vi "禹山溶解氧校准.vi"() -> ()   [LabVIEW 2016, in "斯坦道多参数.lvlib"]
uses:
  <vilib>/Utility/miscctls.llb/LVPointTypeDef.ctl
  <vilib>/Analysis/NI_AALBase.lvlib
  <vilib>/Analysis/NI_AALPro.lvlib
  <vilib>/Utility/config.llb/NI_LVConfig.lvlib
panel:
  out "滤波设定":dbl
  out "第二点信号值":dbl
  out "第一点信号值":dbl
  out "通讯状态":string
  in  "盐度自动获取":bool
  in  "大气压补偿":dbl format="%#.2f"
  in  "盐度补偿":dbl format="%#.2f"
  out "DO %":dbl caption="饱和度值" format="%#.2f"
  out "第二点校准值":dbl
  out "第一点校准值":dbl
  out "最小值":sgl format="%.2g"
  out "最大值":sgl format="%.2g"
  in  "校准停止":bool
  in  "校准模式":u16(ring) items=["两点校准", "单点校准"]
  in  "标液2":dbl
  in  "标液1":dbl
  out "波形图表":dbl(graph) caption="历史曲线"
  out "温度测量值":dbl caption="温度" format="%#.2f"
  out "变异系数":dbl format="%.6g"
  out "standard deviation":dbl caption="标准差" format="%0.2f"
  out "mean":dbl caption="均值" format="%0.2f"
  out "提示":string
  in  "校准启动":bool
  out "DO mg/L":dbl caption="测试值" format="%#.2f"
  out "电极斜率":dbl format="%#.6f"
  out "电极零点":dbl format="%#.6f"
  # "溶解氧电极设定"
  # "℃"
  # "%"
  # "mg/L"
  # "kPa"
  # "请选择校准模式:"
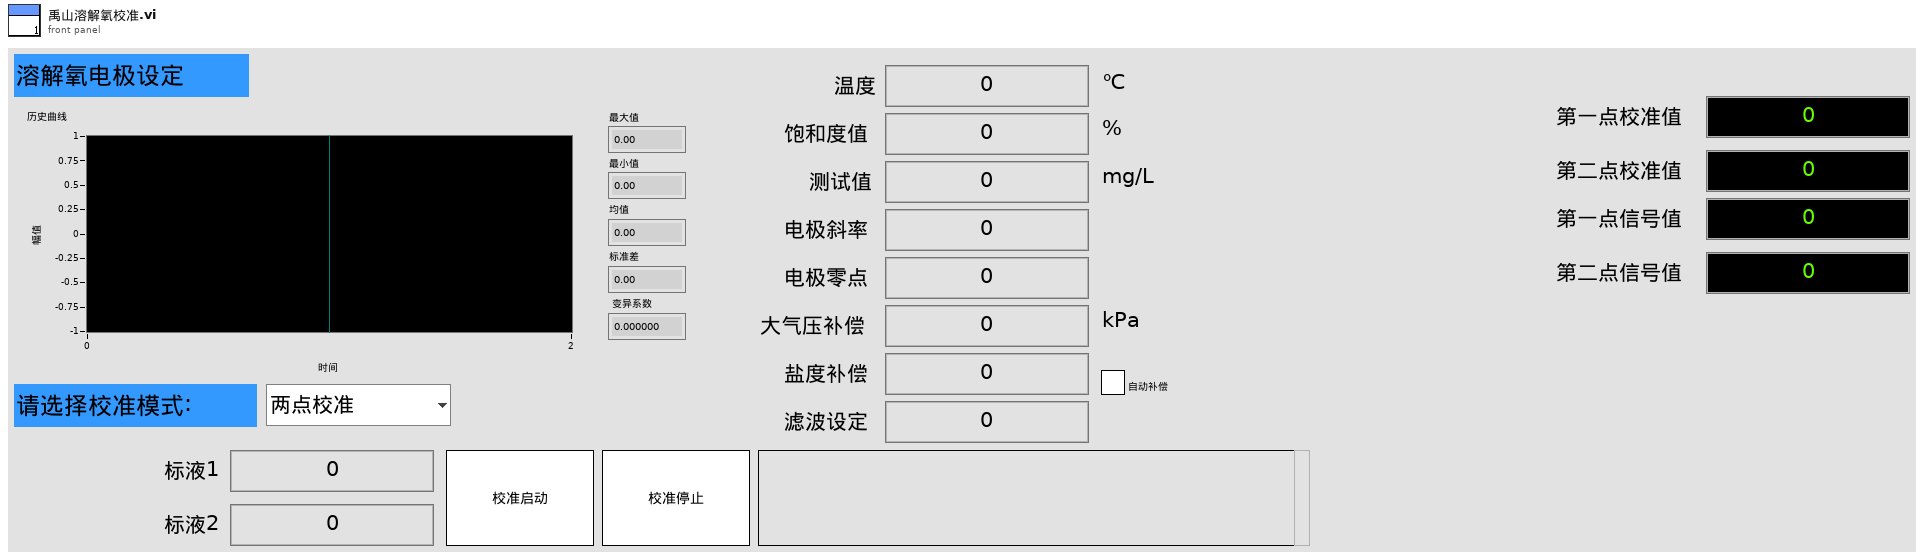
[diagram p1: front panel]
types:
  T1 = enum16{"pH", "DO", "Cond", "Turb", "ORP", "叶绿素a", "藻密度"}
  T2 = typedef "LVPointTypeDef.ctl" = cluster{"Horizontal":i16, "Vertical":i16}
  T3 = cluster{"pH":u32, "DO":u32, "Cond":u32, "Turb":u32, "叶绿素a":u32, "藻密度":u32, "ORP":u32}
  T4 = typedef "NI_LVConfig.lvlib/Config Data RefNum.ctl" = refnum<k1>
  T5 = enum8{"Enabled", "Disabled", "Disabled and Grayed Out"}
  T6 = cluster{"ph":bool, "DO":bool, "Cond":bool, "Turb":bool, "叶绿素a":bool, "藻密度":bool, "ORP":bool}
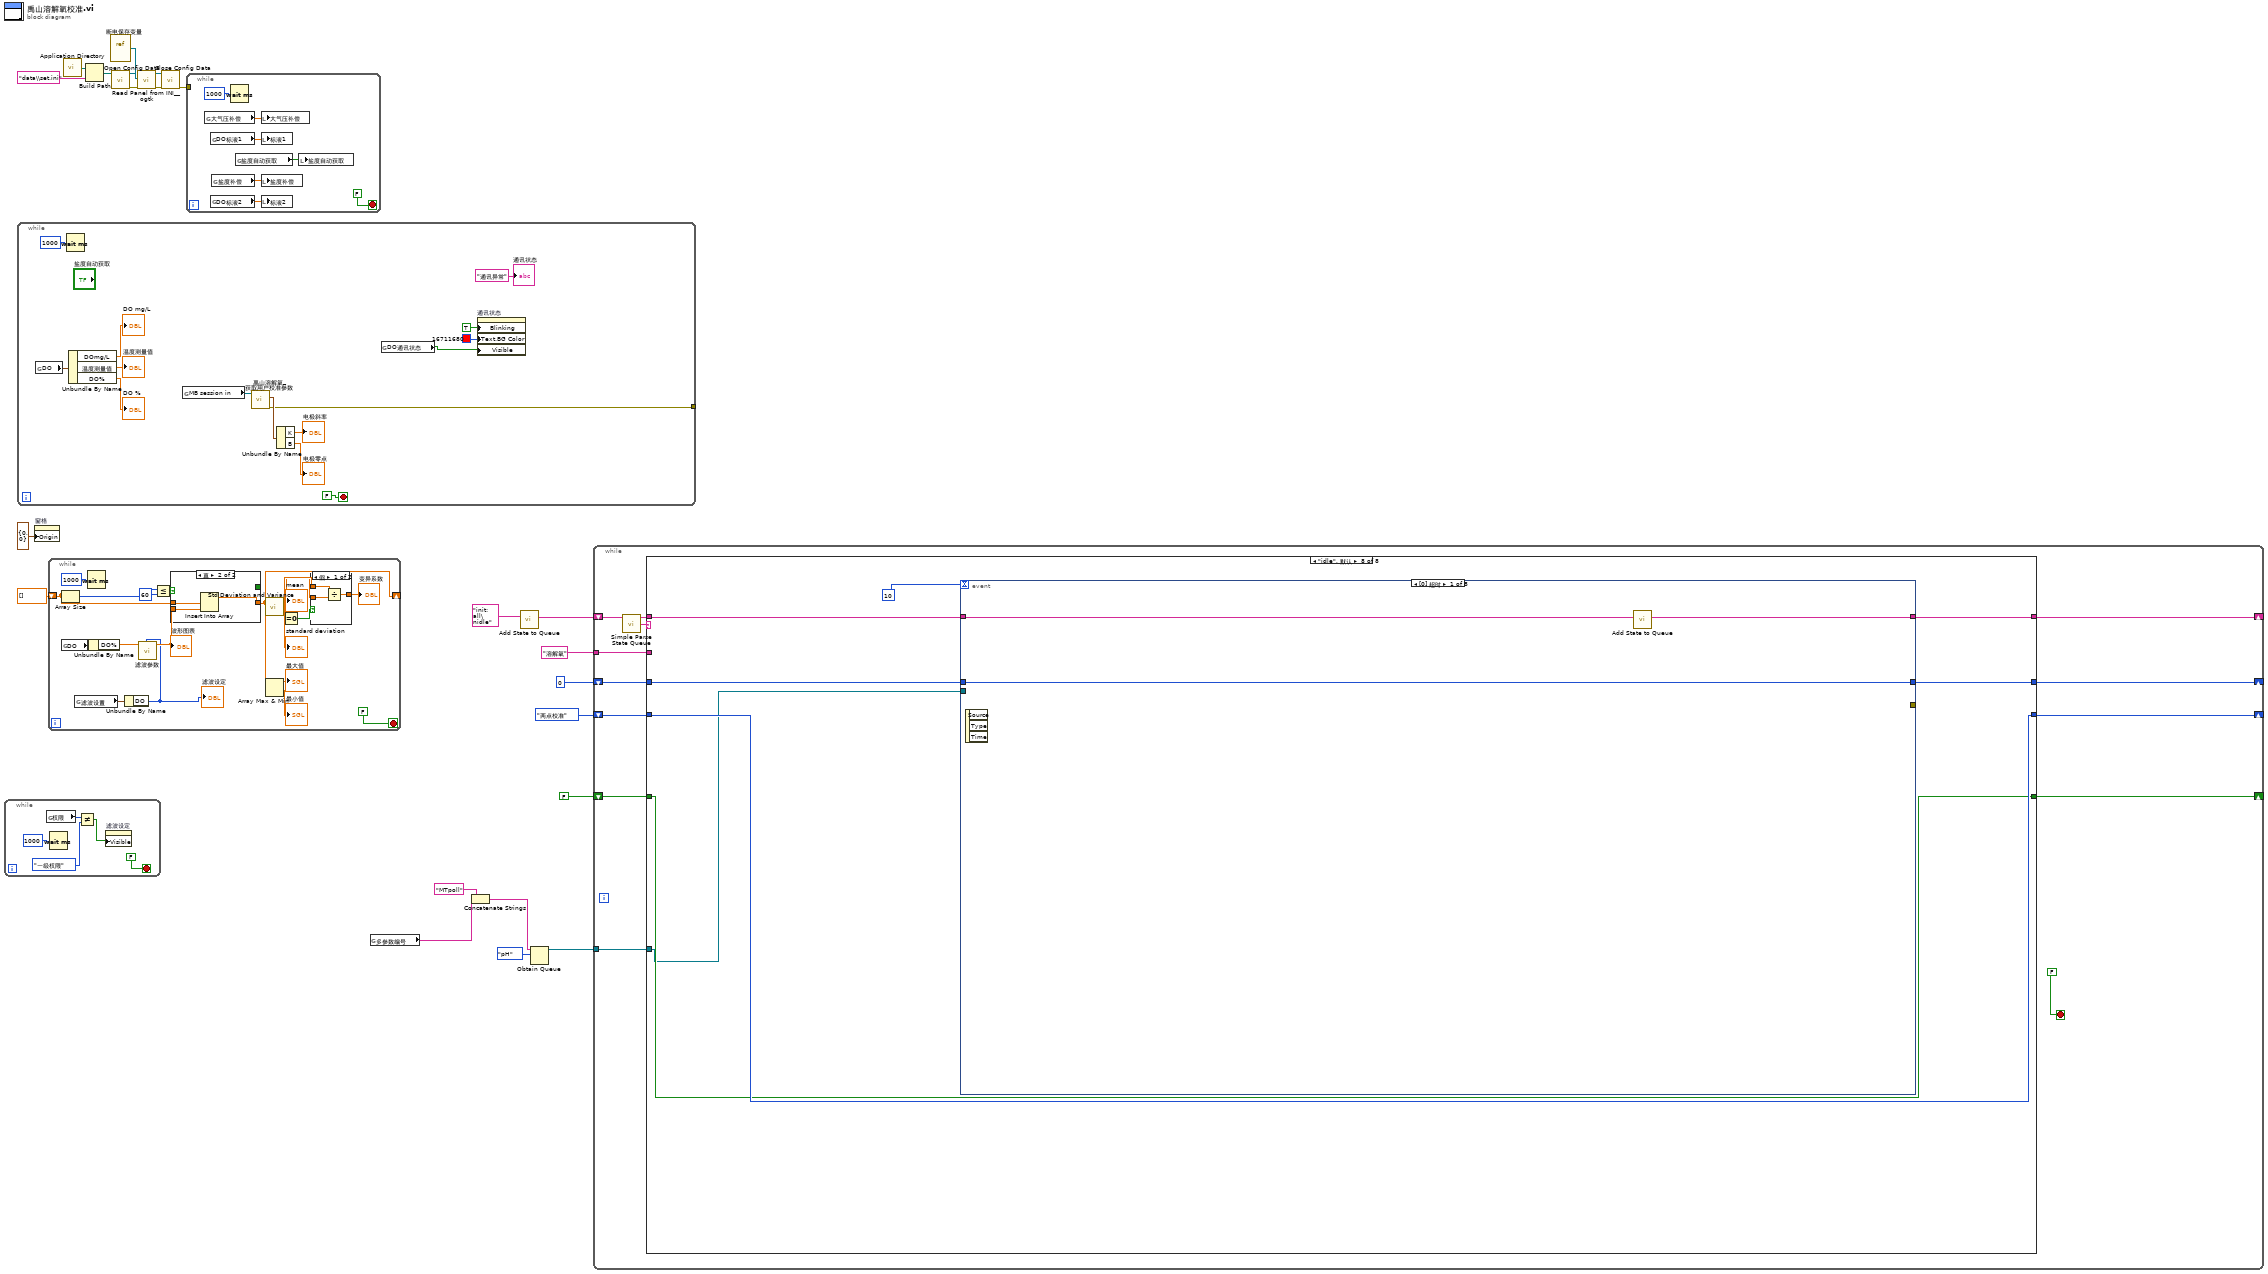
[diagram p0: block diagram]
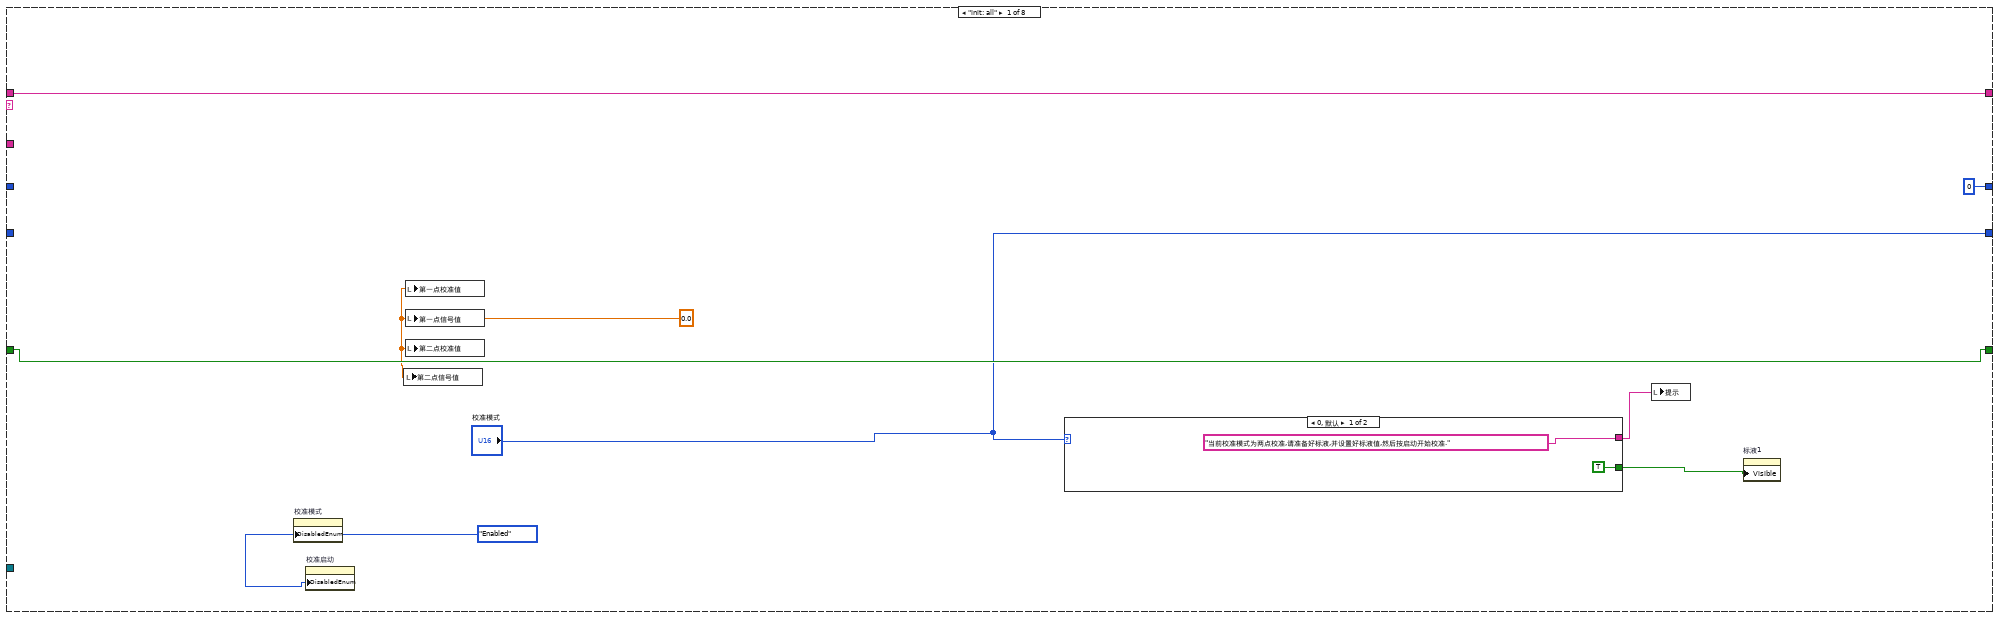
[diagram p2: hidden frame]
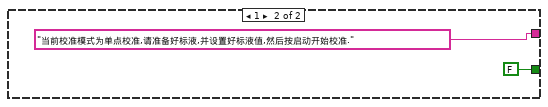
[diagram p3: hidden frame]
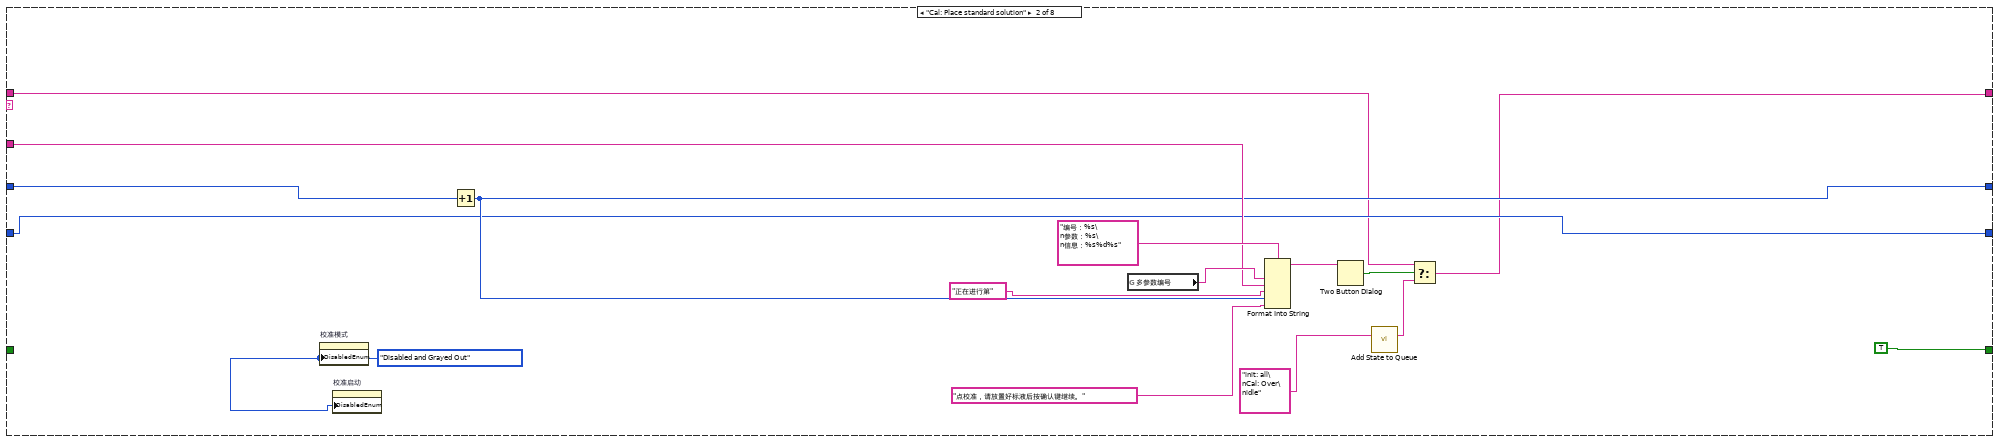
[diagram p4: hidden frame]
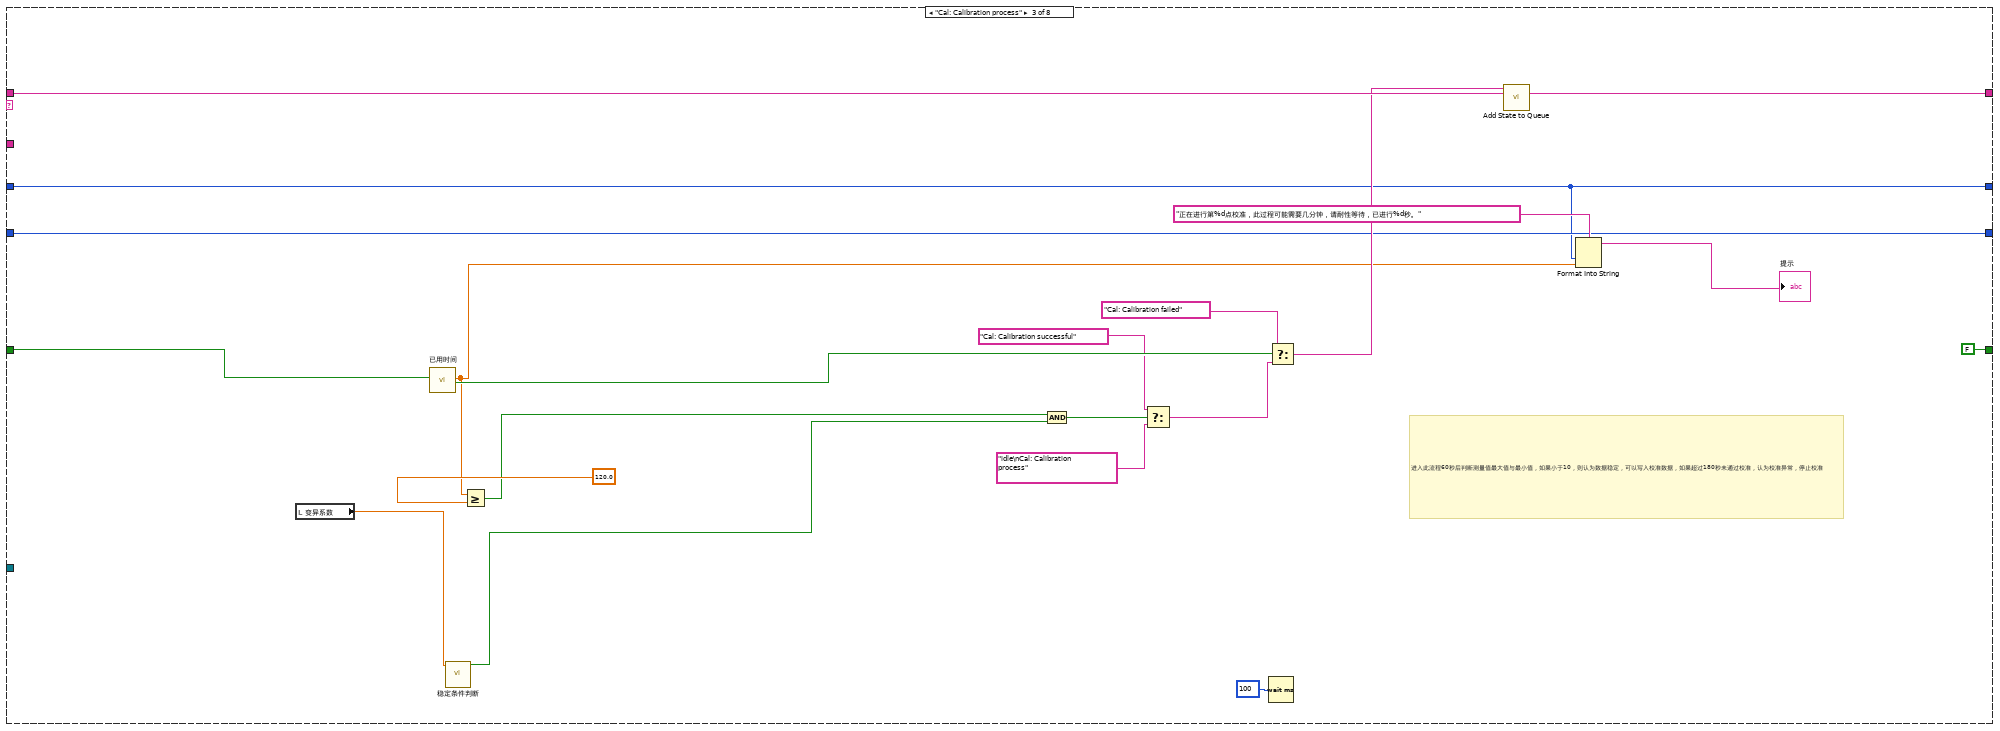
[diagram p5: hidden frame]
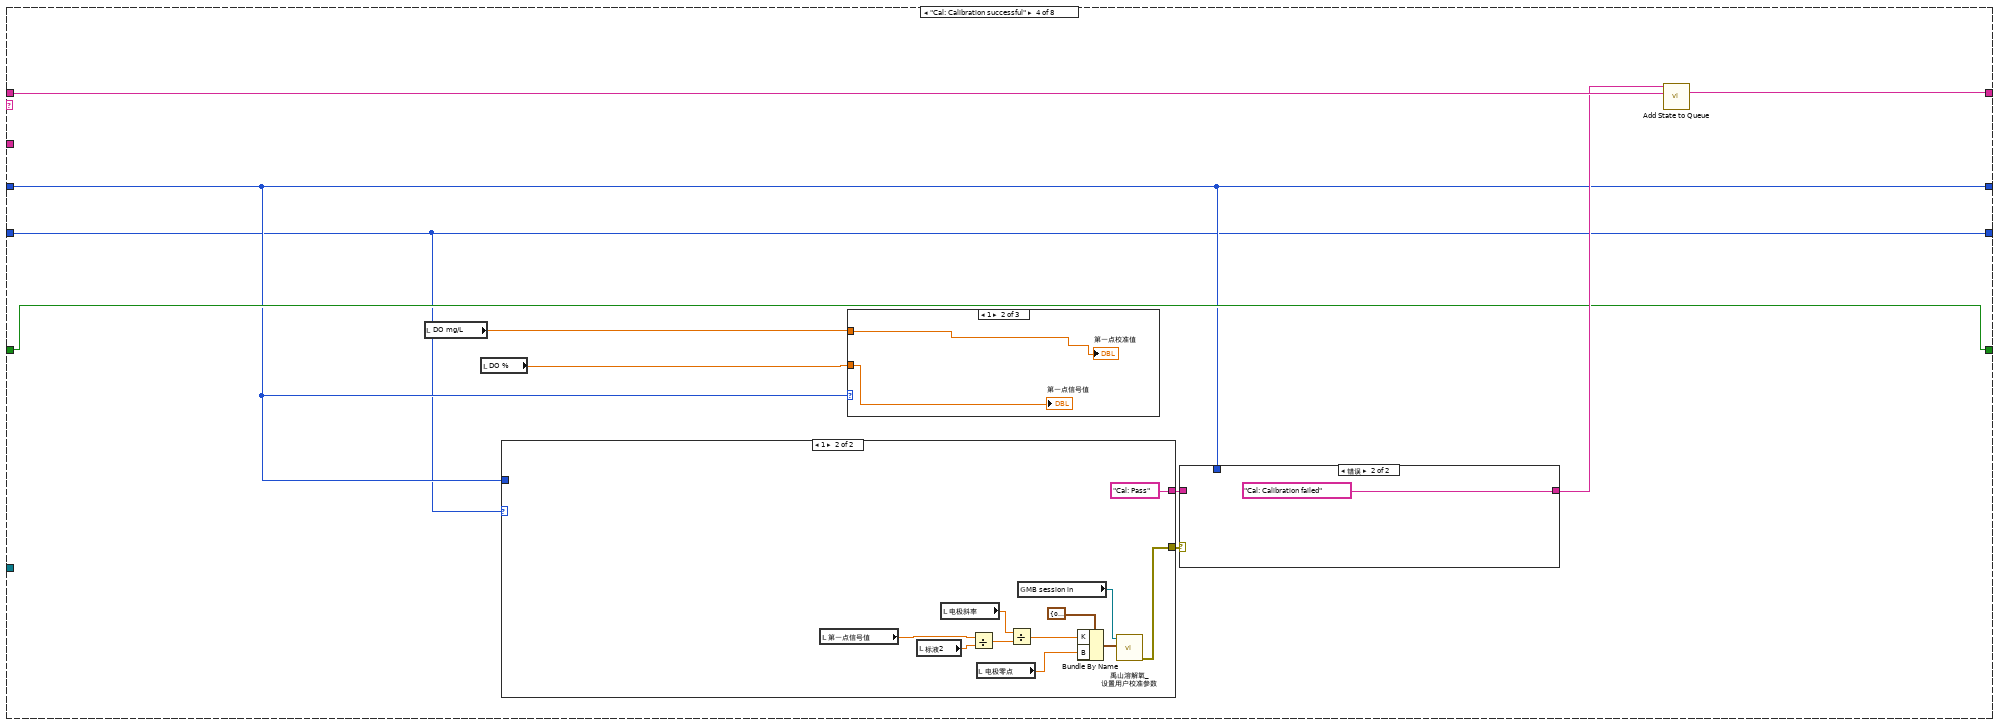
[diagram p6: hidden frame]
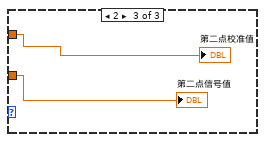
[diagram p8: hidden frame]
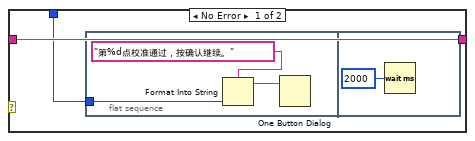
[diagram p9: hidden frame]
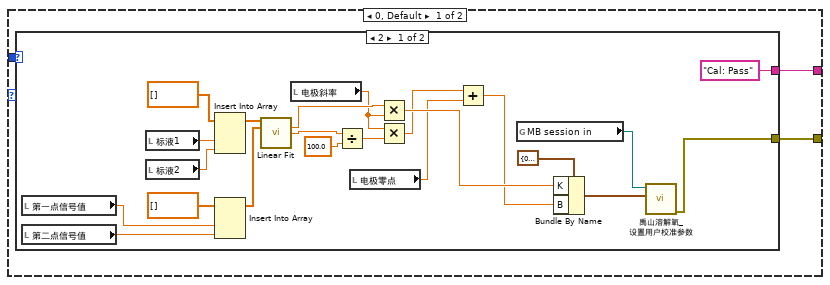
[diagram p10: hidden frame]
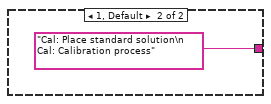
[diagram p11: hidden frame]
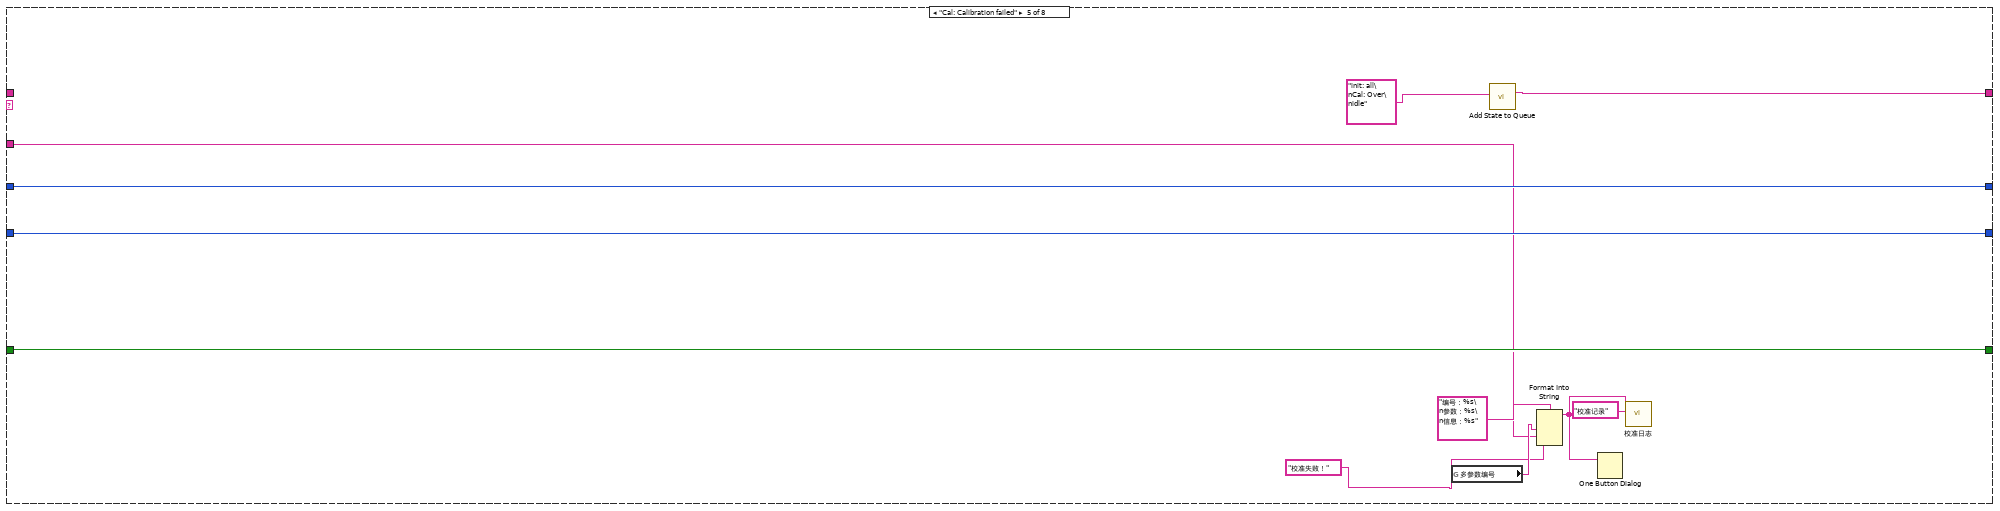
[diagram p12: hidden frame]
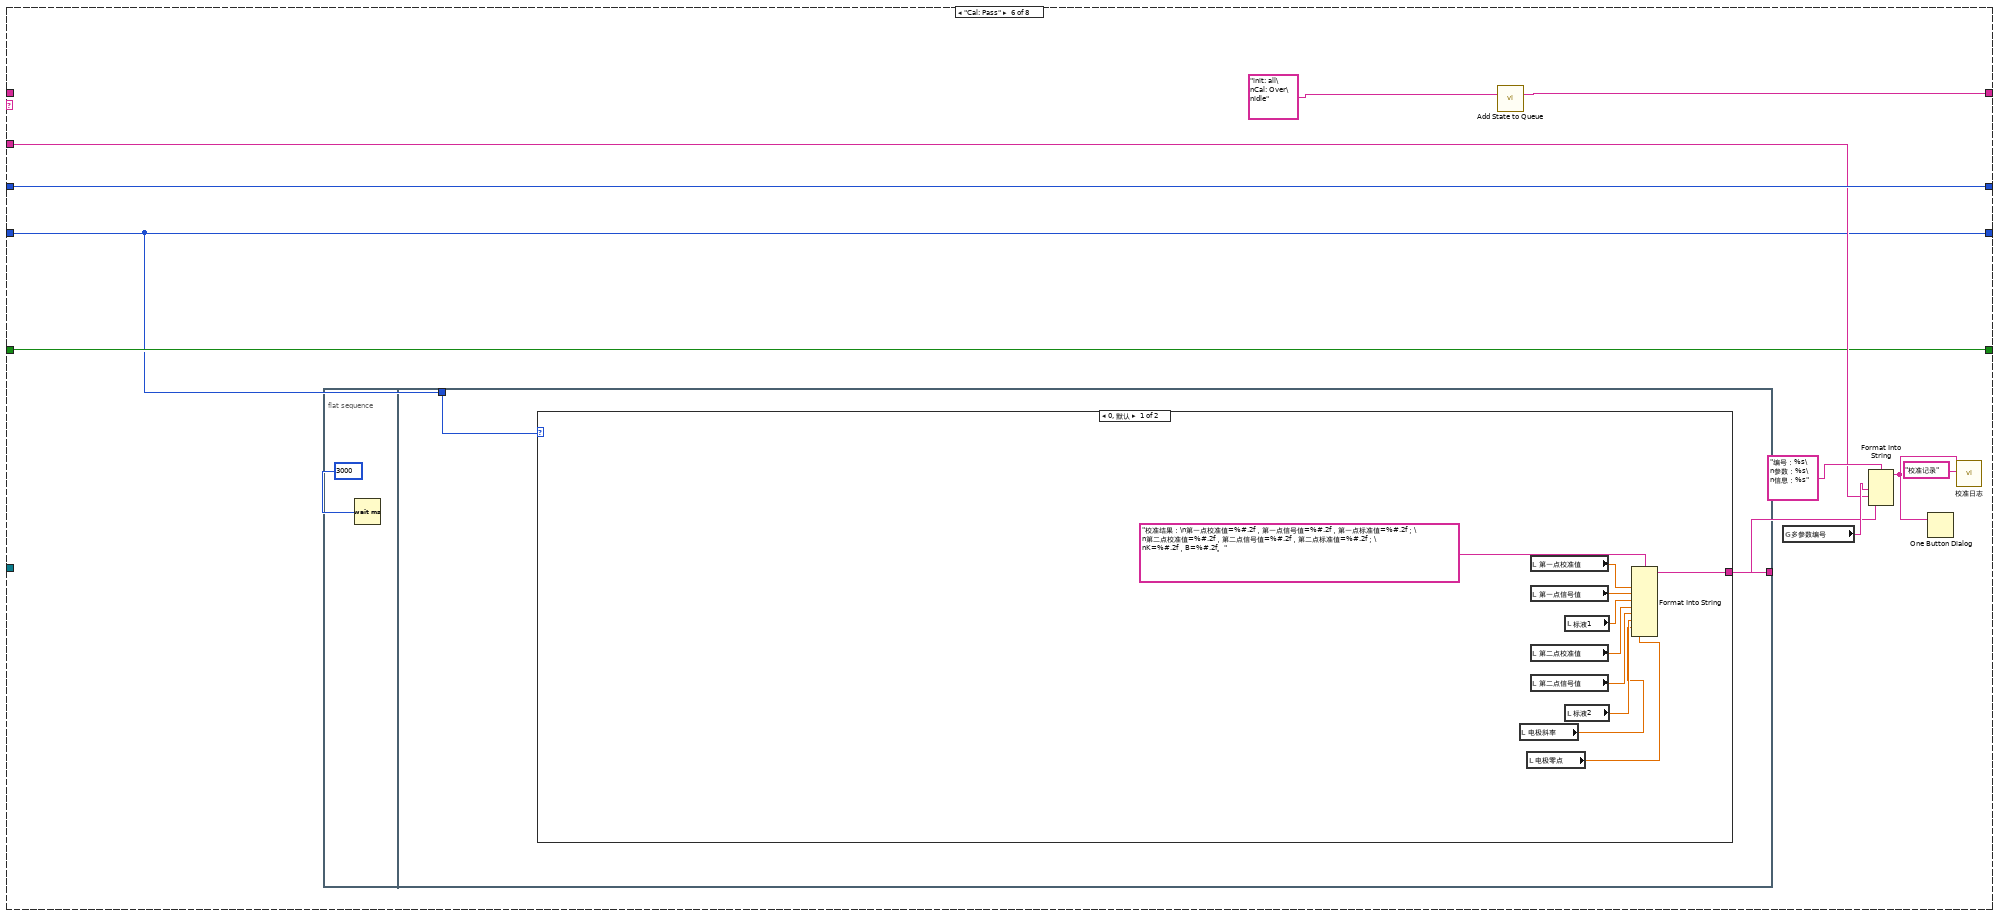
[diagram p13: hidden frame]
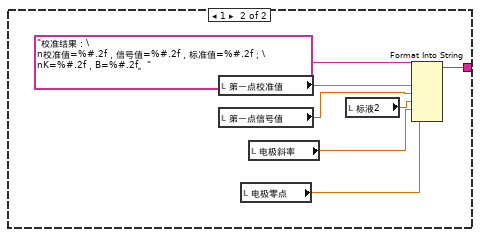
[diagram p14: hidden frame]
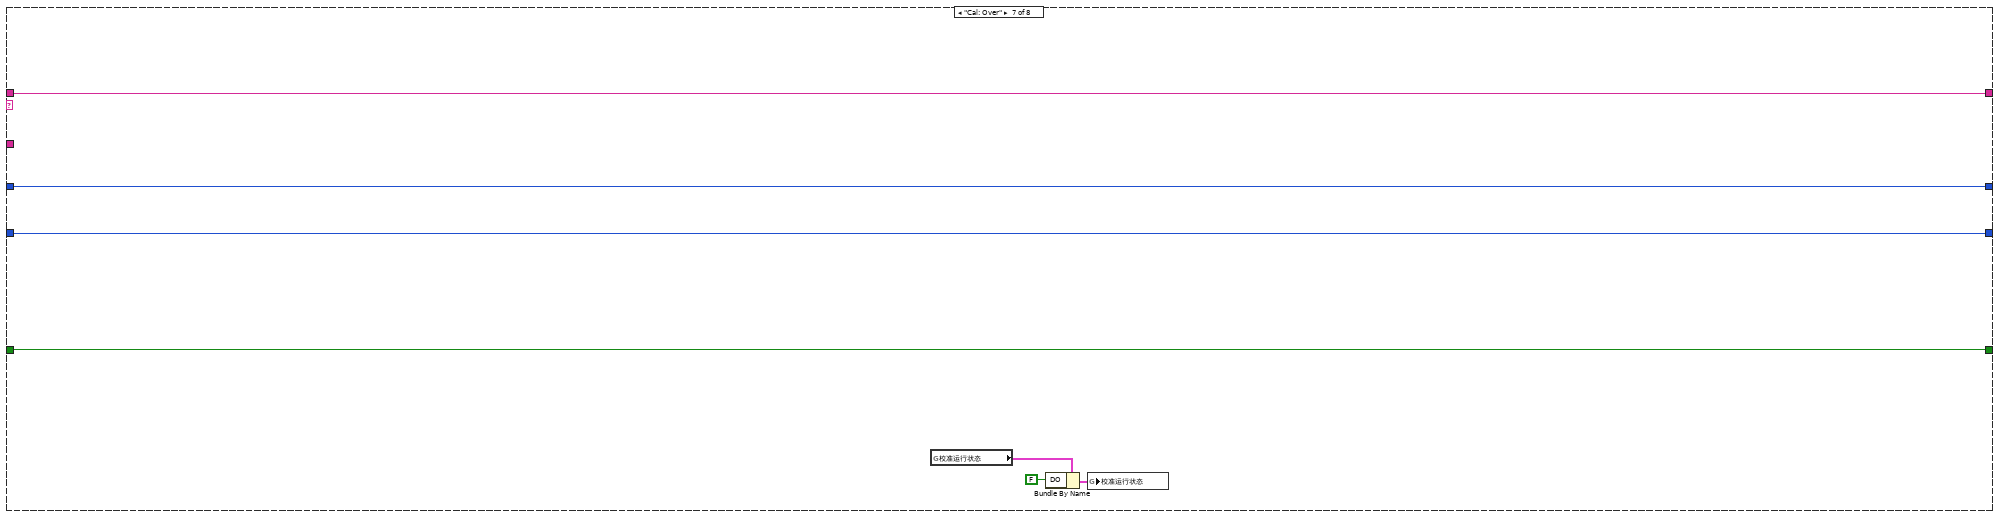
[diagram p15: hidden frame]
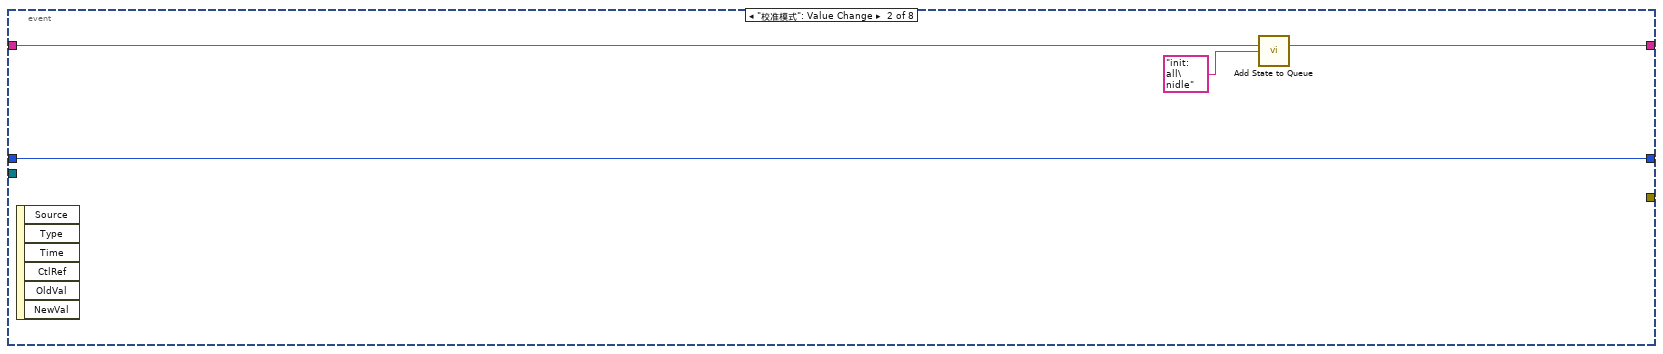
[diagram p16: hidden frame]
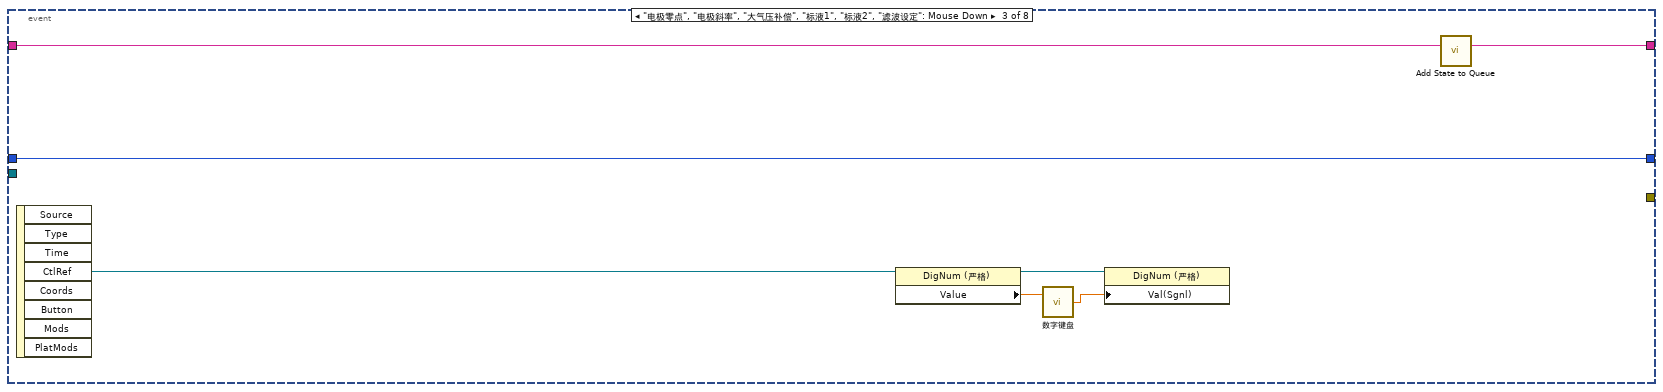
[diagram p17: hidden frame]
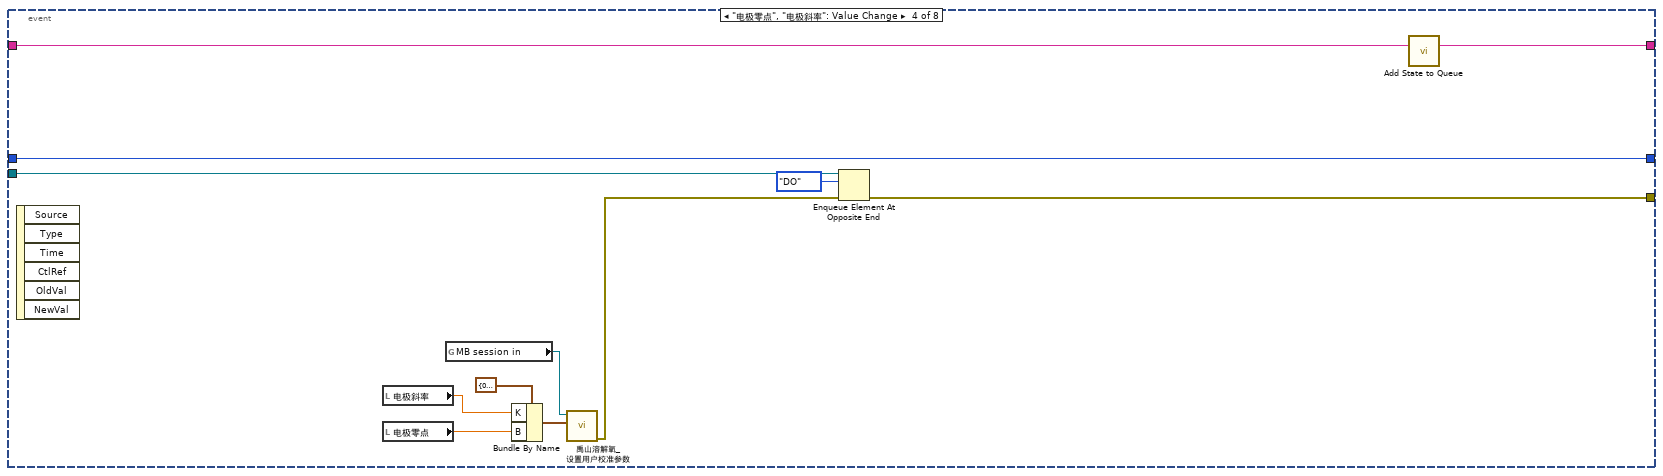
[diagram p18: hidden frame]
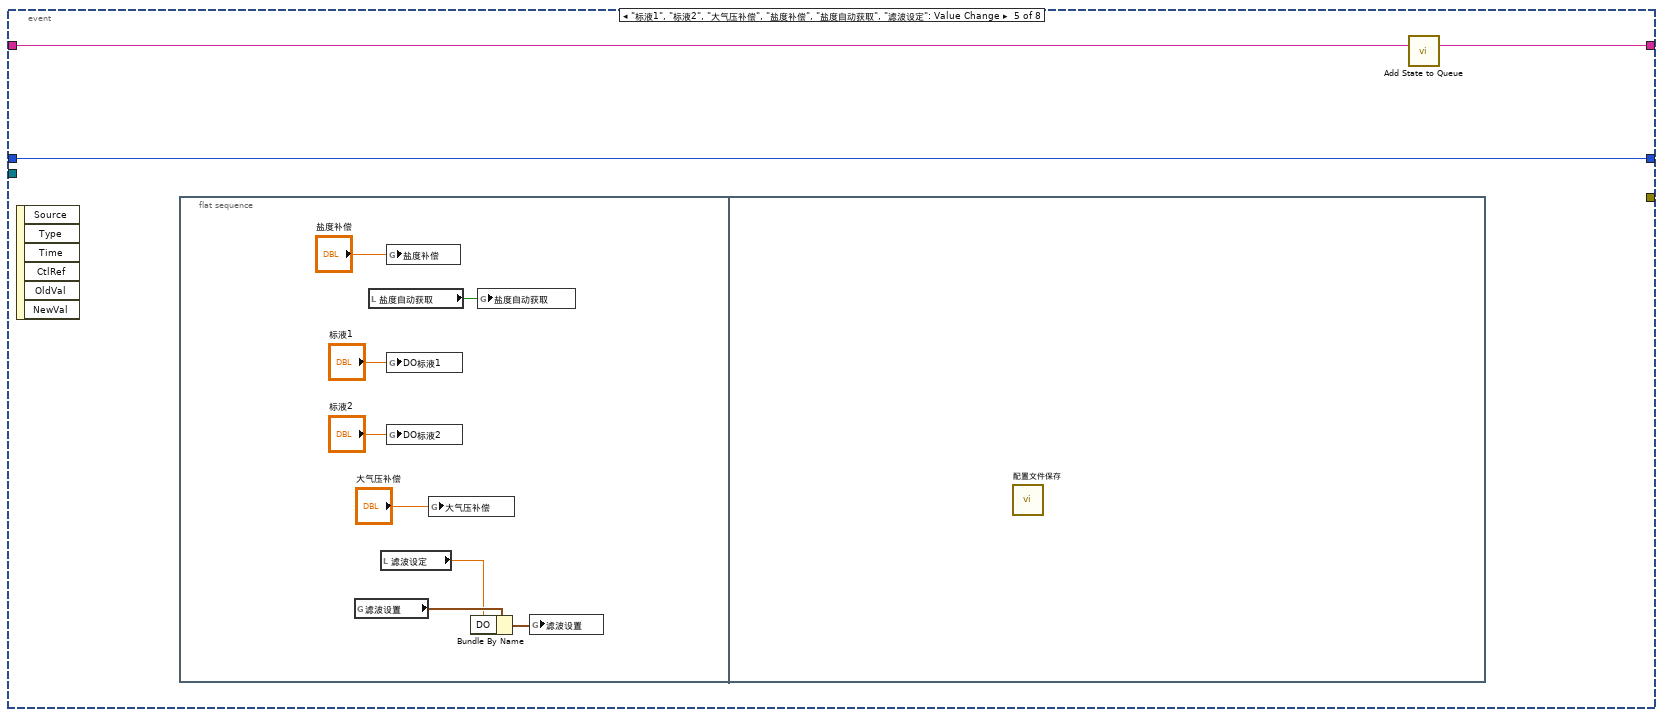
[diagram p19: hidden frame]
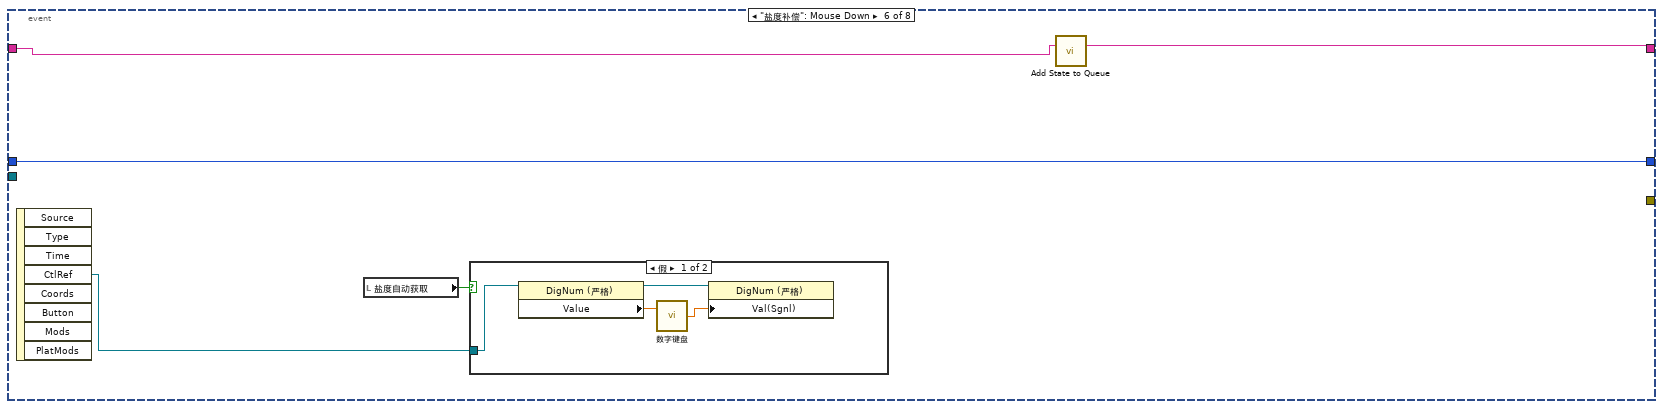
[diagram p20: hidden frame]
diagram:
  n1 = while {
    stop <- FALSE stop-if-true
    n2 = global read "多参数全局变量.vi" "权限"() -> (w26:enum16{"一级权限", "二级权限", "三级权限"})
    n3 = Wait (ms)(milliseconds to wait=u32 1000 ("等待时间（毫秒）")) -> ()  [unwired: 1 out]
    n4 = Not Equal?(x=w26, y=enum16{"一级权限", "二级权限", "三级权限"}."一级权限") -> (x != y?=w23:bool)
    n5 = property on="滤波设定" class="DigNum (严格)"("Visible"=w23) -> ()  [unwired: 2 in, 2 out]
  }
  n6 = while {
    tunnel: [w37] -> _
    stop <- FALSE stop-if-true
    n7 = global read "禹山过程全局变量.vi" "DO"() -> (w34:cluster{"温度测量值":sgl, "DO%":sgl, "DOmg/L":sgl})
    n8 = Wait (ms)(milliseconds to wait=u32 1000 ("等待时间（毫秒）")) -> ()  [unwired: 1 out]
    n9 = Unbundle By Name(w34) -> ("DOmg/L"=→"DO mg/L":sgl, "温度测量值"=→"温度测量值":sgl, "DO%"=→"DO %":sgl)
    n10 = global read "多参数全局变量.vi" "MB session in"() -> (w33:refnum<class "MB_Master.lvclass">)
    n11 = call "禹山溶解氧_获取用户校准参数.vi"("MB session in"=w33) -> ("error out"=w37:errorcluster, "输出值"=w40:cluster{"K":sgl, "B":sgl})  [unwired: 8 in, 1 out]
    n12 = Unbundle By Name(w40) -> ("K"=→"电极斜率":sgl, "B"=→"电极零点":sgl)
    n13 = global read "多参数全局变量.vi" "DO通讯状态"() -> (w28:bool)
    n14 = property on="通讯状态" class="Str"("Blinking"=TRUE ("闪烁"), "Text.BG Color"=u32 16711680, "Visible"=w28) -> ()  [unwired: 2 in, 2 out]
    "通讯状态" <- "通讯异常" ("当前串口")
  }
  n15 = property on="窗格" class="Pane"("Origin"=T2 {"Horizontal"=0, "Vertical"=0} ("原点")) -> ()  [unwired: 2 in, 2 out]
  n16 = while {
    shift-right: [w49] -> _
    shift-left: sgl[] [] -> [w56]
    stop <- FALSE stop-if-true
    n17 = Array Size(array=w56) -> (size(s)=w58:i32)
    n18 = global read "禹山过程全局变量.vi" "DO"() -> (w50:cluster{"温度测量值":sgl, "DO%":sgl, "DOmg/L":sgl})
    n19 = global read "断电保存变量.vi" "滤波设置"() -> (w44:T3)
    n20 = Wait (ms)(milliseconds to wait=u32 1000 ("等待时间（毫秒）")) -> ()  [unwired: 1 out]
    n21 = Unbundle By Name(w50) -> ("DO%"=w46:sgl)
    n22 = Unbundle By Name(w44) -> ("DO"=w43:u32)
    "滤波设定" <- w43
    n23 = call "滤波参数.vi"("滤波次数"=w43, "x"=w46) -> ("mode"=w45:dbl)  [unwired: 9 in]
    "波形图表" <- w45
    n24 = Less Or Equal?(x=w58, y=60) -> (x <= y?=w57:bool)
    n25 = case shown="真" w57 {
      tunnel: w56 -> [w69 w72]
      tunnel: w45 -> [w67 w71]
      tunnel: [w65 w70] -> w49
      tunnel: [TRUE _] -> _
      frame False {
        n26 = Replace Array Subset(array=w69, new element=w67) -> (w68:sgl[])  [unwired: 1 in]
        n27 = Rotate 1D Array(1:w68, 2:-1 ("n")) -> (0:w65:sgl[])
      }
      frame True {
        n28 = Insert Into Array(array=w72, new element=w71) -> (w70:sgl[])  [unwired: 1 in]
      }
    }
    n29 = call <vilib>:"Std Deviation and Variance.vi"("X"=w49) -> ("mean"=w51:dbl, "standard deviation"=w52:dbl)  [unwired: 1 in, 1 out]
    "standard deviation" <- w52
    "mean" <- w51
    n30 = Array Max & Min(array=w49) -> (max value=→"最大值":sgl, min value=→"最小值":sgl)  [unwired: 2 out]
    n31 = Equal To 0?(x=w51) -> (x = 0?=w55:bool)
    n32 = case shown="假" w55 {
      tunnel: w52 -> [w63 _]
      tunnel: [w62 _] -> w54
      tunnel: w51 -> [w61 _]
      frame False {
        n33 = Divide(x=w63, y=w61) -> (x/y=w62:dbl)
      }
      frame True {
      }
    }
    "变异系数" <- w54
  }
  n34 = call <vilib>:"Application Directory.vi"() -> ("Application Directory"=w17:path)
  n35 = Build Path(base path=w17, name or relative path="data\\set.ini" ("名称或相对路径")) -> (appended path=w18:path)
  n36 = vi-ref "断电保存变量.vi"() -> (w20:refnum<vi>)
  n37 = call <vilib>:"Open Config Data.vi"("configuration file path"=w18) -> ("error out"=w14:errorcluster, "refnum"=w13:T4)  [unwired: 8 in, 1 out]
  n38 = call <userlib>:"Read Panel from INI__ogtk.vi"("error in (no error)"=w14, "VI ref"=w20, "refnum"=w13) -> ("error out"=w16:errorcluster, "refnum out"=w15:T4)  [unwired: 7 in]
  n39 = call <vilib>:"Close Config Data.vi"("error in (no error)"=w16, "refnum"=w15) -> ("error out"=w12:errorcluster)  [unwired: 8 in, 1 out]
  n40 = while {
    tunnel: w12 -> [_]
    stop <- FALSE stop-if-true
    n41 = global read "断电保存变量.vi" "大气压补偿"() -> (w75:dbl)
    n42 = global read "断电保存变量.vi" "DO标液1"() -> (w77:dbl)
    n43 = global read "断电保存变量.vi" "DO标液2"() -> (w76:dbl)
    n44 = global read "断电保存变量.vi" "盐度补偿"() -> (w73:dbl)
    n45 = Wait (ms)(milliseconds to wait=u32 1000 ("等待时间（毫秒）")) -> ()  [unwired: 1 out]
    n46 = global read "断电保存变量.vi" "盐度自动获取"() -> (w74:bool)
    n47 = local write "大气压补偿"(w75) -> ()
    n48 = local write "标液1"(w77) -> ()
    n49 = local write "盐度补偿"(w73) -> ()
    n50 = local write "标液2"(w76) -> ()
    n51 = local write "盐度自动获取"(w74) -> ()
  }
  n52 = global read "多参数全局变量.vi" "多参数编号"() -> (w2:string)
  n53 = Concatenate Strings("MTpoll" ("名称（未命名）"), w2) -> (w4:string)
  n54 = call "Add State to Queue.vi"("State(s) In (\"\")"="init: all\nidle" ("State(s) In (\"\")")) -> ("States Out"=w10:string)  [unwired: 14 in]
  n55 = Obtain Queue(name (unnamed)=w4, element data type=T1."pH" ("枚举")) -> (queue out=w1:refnum<queue>)  [unwired: 3 in, 2 out]
  n56 = while {
    shift-right: [w88] -> _
    shift-left: w10 -> [w92]
    shift-right: [w85] -> _
    shift-left: 0 -> [w87]
    tunnel: "溶解氧" ("State(s) In (\"\")") -> [w86]
    shift-right: [w83] -> _
    shift-left: enum16{"两点校准", "单点校准"}."两点校准" ("校准模式") -> [w84]
    shift-right: [w81] -> _
    shift-left: FALSE -> [w82]
    tunnel: w1 -> [w80]
    stop <- FALSE stop-if-true
    n57 = call "Simple Parse State Queue.vi"("State Queue"=w92) -> ("Remain States"=w89:string, "Next State"=w90:string)  [unwired: 13 in]
    n58 = case shown="\"idle\", 默认" w90 {
      tunnel: w89 -> [w100 w108 w140 w149 _ _ w248 w256]
      tunnel: [w100 w107 w139 w148 w207 w212 w248 w255] -> w88
      tunnel: w87 -> [_ w116 w125 w143 w210 w221 w247 w253]
      tunnel: w86 -> [_ w117 _ _ w201 w217 _ _]
      tunnel: [0 w114 w125 w143 w210 w221 w247 w254] -> w85
      tunnel: w84 -> [_ w113 w126 w142 w209 w213 w246 w252]
      tunnel: ["校准模式" w113 w126 w142 w209 w213 w246 w252] -> w83
      tunnel: w82 -> [w97 _ w128 w144 w208 w216 w245 w250]
      tunnel: [w97 TRUE FALSE w144 w208 w216 w245 w250] -> w81
      tunnel: w80 -> [_ _ _ _ _ _ _ w249]
      frame "init: all" {
        w95 = T5."Enabled" ("禁用")
        w96 = 0.0 ("第一点校准值")
        n59 = property on="校准模式" class="Ring (严格)"("DisabledEnum"=w95) -> ()  [unwired: 2 in, 2 out]
        n60 = property on="校准启动" class="Bool"("DisabledEnum"=w95) -> ()  [unwired: 2 in, 2 out]
        n61 = local write "第二点信号值"(w96) -> ()
        n62 = local write "第一点校准值"(w96) -> ()
        n63 = local write "第一点信号值"(w96) -> ()
        n64 = local write "第二点校准值"(w96) -> ()
        n65 = case shown="0, 默认" "校准模式" {
          tunnel: ["当前校准模式为两点校准,请准备好标液,并设置好标液值,然后按启动开始校准." ("提示") "当前校准模式为单点校准,请准备好标液,并设置好标液值,然后按启动开始校准." ("提示")] -> w99
          tunnel: [TRUE ("可见") FALSE ("可见")] -> w93
          frame 0, Default {
          }
          frame 1 {
          }
        }
        n66 = local write "提示"(w99) -> ()
        n67 = property on="标液1" class="DigNum (严格)"("Visible"=w93) -> ()  [unwired: 2 in, 2 out]
      }
      frame "Cal: Place standard solution" {
        w106 = T5."Disabled and Grayed Out" ("禁用")
        n68 = property on="校准模式" class="Ring (严格)"("DisabledEnum"=w106) -> ()  [unwired: 2 in, 2 out]
        n69 = property on="校准启动" class="Bool"("DisabledEnum"=w106) -> ()  [unwired: 2 in, 2 out]
        n70 = Increment(x=w116) -> (x+1=w114:i32)
        n71 = global read "多参数全局变量.vi" "多参数编号"() -> (w119:string)
        n72 = Format Into String(format string="编号：%s\n参数：%s\n信息：%s%d%s" ("格式字符串"), w119, w117, "正在进行第" ("消息"), w114, "点校准，请放置好标液后按确认键继续。" ("消息")) -> (resulting string=w111:string)  [unwired: 2 in, 1 out]
        n73 = Two Button Dialog(message=w111) -> (T button?=w110:bool)  [unwired: 2 in]
        n74 = call "Add State to Queue.vi"("State(s) In (\"\")"="init: all\nCal: Over\nidle" ("State(s) In (\"\")")) -> ("States Out"=w109:string)  [unwired: 14 in]
        n75 = Select(t=w108, s=w110, f=w109) -> (s? t:f=w107:string)
      }
      frame "Cal: Calibration process" {
        # "进入此流程60秒后判断测量值最大值与最小值，如果小于10，则认为数据稳定，可以写入校准数据，如果超过180秒未通过校准，认为校准异常，停止校准"
        n76 = local read "变异系数"() -> (w122:dbl)
        n77 = call "已用时间"("Reset"=w128) -> ("Elapsed Time (s)"=w124:dbl, "Time has Elapsed"=w141:bool)  [unwired: 11 in, 6 out]
        n78 = call "稳定条件判断.vi"("变异系数"=w122) -> ("布尔"=w121:bool)  [unwired: 10 in]
        n79 = Greater Or Equal?(x=w124, y=120.0) -> (x >= y?=w136:bool)
        n80 = And(x=w136, y=w121) -> (x .and. y?=w133:bool)
        n81 = Select(t="Cal: Calibration successful" ("State(s) In (\"\")"), s=w133, f="idle\nCal: Calibration process" ("State(s) In (\"\")")) -> (s? t:f=w132:string)
        n82 = Wait (ms)(milliseconds to wait=u32 100 ("等待时间（毫秒）")) -> ()  [unwired: 1 out]
        n83 = Select(t="Cal: Calibration failed" ("State(s) In (\"\")"), s=w141, f=w132) -> (s? t:f=w131:string)
        n84 = call "Add State to Queue.vi"("State(s) In Front (\"\")"=w131, "State(s) In (\"\")"=w140) -> ("States Out"=w139:string)  [unwired: 13 in]
        n85 = Format Into String(format string="正在进行第%d点校准，此过程可能需要几分钟，请耐性等待，已进行%d秒。" ("格式字符串"), w125, w124) -> (resulting string=→"提示":string)  [unwired: 2 in, 1 out]
      }
      frame "Cal: Calibration successful" {
        n86 = local read "DO mg/L"() -> (w145:dbl)
        n87 = local read "DO %"() -> (w146:dbl)
        n88 = case shown="1" w142 {
          tunnel: [w165 w189] -> w151
          tunnel: [w164 "Cal: Pass" ("State(s) In (\"\")")] -> w150
          tunnel: w143 -> [w163 _]
          frame 0, Default {
            n89 = case shown="2" w163 {
              tunnel: [w166 _] -> w165
              tunnel: ["Cal: Pass" ("State(s) In (\"\")") "Cal: Place standard solution\n Cal: Calibration process" ("State(s) In (\"\")")] -> w164
              frame 2 {
                n90 = local read "第一点信号值"() -> (w185:dbl)
                n91 = local read "第二点信号值"() -> (w184:dbl)
                n92 = local read "标液1"() -> (w182:dbl)
                n93 = local read "标液2"() -> (w181:dbl)
                n94 = Insert Into Array(array=dbl[] [] ("Weight"), new element #1=w182, new element #2=w181) -> (w180:dbl[])  [unwired: 1 in]
                n95 = Insert Into Array(array=dbl[] [] ("Weight"), new element #1=w185, new element #2=w184) -> (w179:dbl[])  [unwired: 1 in]
                n96 = call <vilib>:"Linear Fit.vi"("Y"=w180, "X"=w179) -> ("slope"=w175:dbl, "intercept"=w172:dbl)  [unwired: 9 in, 3 out]
                n97 = local read "电极斜率"() -> (w173:dbl)
                n98 = Divide(x=w172, y=100.0) -> (x/y=w168:dbl)
                n99 = local read "电极零点"() -> (w170:dbl)
                n100 = Multiply(x=w175, y=w173) -> (x*y=w174:dbl)
                n101 = Multiply(x=w173, y=w168) -> (x*y=w171:dbl)
                n102 = Add(x=w171, y=w170) -> (x+y=w169:dbl)
                n103 = global read "多参数全局变量.vi" "MB session in"() -> (w178:refnum<class "MB_Master.lvclass">)
                n104 = Bundle By Name(cluster=cluster{"K":sgl, "B":sgl} {"K"=0.0, "B"=0.0} ("用户校准参数"), "K"=w174, "B"=w169) -> (w177:cluster{"K":sgl, "B":sgl})
                n105 = call "禹山溶解氧_设置用户校准参数.vi"("用户校准参数"=w177, "MB session in"=w178) -> ("error out"=w166:errorcluster)  [unwired: 8 in, 1 out]
              }
              frame 1, Default {
              }
            }
          }
          frame 1 {
            n106 = local read "第一点信号值"() -> (w194:dbl)
            n107 = local read "标液2"() -> (w193:dbl)
            n108 = local read "电极斜率"() -> (w191:dbl)
            n109 = Divide(x=w194, y=w193) -> (x/y=w190:dbl)
            n110 = local read "电极零点"() -> (w195:dbl)
            n111 = Divide(x=w191, y=w190) -> (x/y=w192:dbl)
            n112 = global read "多参数全局变量.vi" "MB session in"() -> (w198:refnum<class "MB_Master.lvclass">)
            n113 = Bundle By Name(cluster=cluster{"K":sgl, "B":sgl} {"K"=0.0, "B"=0.0} ("用户校准参数"), "K"=w192, "B"=w195) -> (w197:cluster{"K":sgl, "B":sgl})
            n114 = call "禹山溶解氧_设置用户校准参数.vi"("用户校准参数"=w197, "MB session in"=w198) -> ("error out"=w189:errorcluster)  [unwired: 8 in, 1 out]
          }
        }
        n115 = case shown="1" w143 {
          tunnel: w146 -> [_ w153 w155]
          tunnel: w145 -> [_ w152 w154]
          frame 0, Default {
          }
          frame 1 {
            "第一点信号值" <- w153
            "第一点校准值" <- w152
          }
          frame 2 {
            "第二点信号值" <- w155
            "第二点校准值" <- w154
          }
        }
        n116 = case shown="错误" w151 {
          tunnel: w150 -> [w157 _]
          tunnel: [w157 "Cal: Calibration failed" ("State(s) In (\"\")")] -> w147
          tunnel: w143 -> [w156 _]
          frame No Error {
            n117 = flat-sequence {
              tunnel: w156 -> [w158]
              frame #0 {
                n118 = Format Into String(format string="第%d点校准通过，按确认继续。" ("格式字符串"), w158) -> (resulting string=w160:string)  [unwired: 2 in, 1 out]
                n119 = One Button Dialog(message=w160) -> ()  [unwired: 1 in, 1 out]
              }
              frame #1 {
                n120 = Wait (ms)(milliseconds to wait=u32 2000 ("等待时间（毫秒）")) -> ()  [unwired: 1 out]
              }
            }
          }
          frame Error {
          }
        }
        n121 = call "Add State to Queue.vi"("State(s) In Front (\"\")"=w147, "State(s) In (\"\")"=w149) -> ("States Out"=w148:string)  [unwired: 13 in]
      }
      frame "Cal: Calibration failed" {
        n122 = global read "多参数全局变量.vi" "多参数编号"() -> (w204:string)
        n123 = call "Add State to Queue.vi"("State(s) In (\"\")"="init: all\nCal: Over\nidle" ("State(s) In (\"\")")) -> ("States Out"=w207:string)  [unwired: 14 in]
        n124 = Format Into String(format string="编号：%s\n参数：%s\n信息：%s" ("格式字符串"), w204, w201, "校准失败！" ("消息")) -> (resulting string=w203:string)  [unwired: 2 in, 1 out]
        n125 = One Button Dialog(message=w203) -> ()  [unwired: 1 in, 1 out]
        n126 = call "校准日志.vi"("table"="校准记录", "日志信息"=w203) -> ()  [unwired: 9 in, 1 out]
      }
      frame "Cal: Pass" {
        n127 = flat-sequence {
          tunnel: [w224] -> w214
          tunnel: w213 -> [w223]
          frame #0 {
            n128 = Wait (ms)(milliseconds to wait=u32 3000 ("等待时间（毫秒）")) -> ()  [unwired: 1 out]
          }
          frame #1 {
            n129 = case shown="0, 默认" w223 {
              tunnel: [w234 w241] -> w224
              frame 0, Default {
                n130 = local read "电极斜率"() -> (w226:dbl)
                n131 = local read "电极零点"() -> (w225:dbl)
                n132 = local read "第一点校准值"() -> (w232:dbl)
                n133 = local read "第一点信号值"() -> (w233:dbl)
                n134 = local read "第二点校准值"() -> (w229:dbl)
                n135 = local read "第二点信号值"() -> (w228:dbl)
                n136 = local read "标液1"() -> (w230:dbl)
                n137 = local read "标液2"() -> (w227:dbl)
                n138 = Format Into String(format string="校准结果：\n第一点校准值=%#.2f，第一点信号值=%#.2f，第一点标准值=%#.2f；\n第二点校准值=%#.2f，第二点信号值=%#.2f，第二点标准值=%#.2f；\nK=%#.2f，B=%#.2f。" ("提示"), w232, w233, w230, w229, w228, w227, w226, w225) -> (resulting string=w234:string)  [unwired: 2 in, 1 out]
              }
              frame 1 {
                n139 = local read "第一点校准值"() -> (w240:dbl)
                n140 = local read "第一点信号值"() -> (w238:dbl)
                n141 = local read "电极零点"() -> (w235:dbl)
                n142 = local read "电极斜率"() -> (w236:dbl)
                n143 = local read "标液2"() -> (w237:dbl)
                n144 = Format Into String(format string="校准结果：\n校准值=%#.2f，信号值=%#.2f，标准值=%#.2f；\nK=%#.2f，B=%#.2f。" ("提示"), w240, w238, w237, w236, w235) -> (resulting string=w241:string)  [unwired: 2 in, 1 out]
              }
            }
          }
        }
        n145 = call "Add State to Queue.vi"("State(s) In (\"\")"="init: all\nCal: Over\nidle" ("State(s) In (\"\")")) -> ("States Out"=w212:string)  [unwired: 14 in]
        n146 = global read "多参数全局变量.vi" "多参数编号"() -> (w218:string)
        n147 = Format Into String(format string="编号：%s\n参数：%s\n信息：%s" ("格式字符串"), w218, w217, w214) -> (resulting string=w215:string)  [unwired: 2 in, 1 out]
        n148 = One Button Dialog(message=w215) -> ()  [unwired: 1 in, 1 out]
        n149 = call "校准日志.vi"("table"="校准记录", "日志信息"=w215) -> ()  [unwired: 9 in, 1 out]
      }
      frame "Cal: Over" {
        n150 = global read "多参数全局变量.vi" "校准运行状态"() -> (w243:T6)
        n151 = Bundle By Name(cluster=w243, "DO"=FALSE) -> (w244:T6)
        n152 = global write "多参数全局变量.vi" "校准运行状态"(w244) -> ()
      }
      frame "idle", Default {
        n153 = event shown="[0] 超时" {
          selector: _ -> [_ _ _ _ _ _ _ _]
          dyn-events: _ -> [_ _ _ _ _ _ _ _]
          timeout: 10 -> [_ _ _ _ _ _ _ _]
          tunnel: [_ _ _ w273 _ _ _ _] -> _
          tunnel: w256 -> [w259 w263 w268 w274 w283 w294 w309 _]
          tunnel: [w258 w262 w269 w281 w284 w296 w308 w311] -> w255
          tunnel: [w257 w260 w270 w282 w285 w295 w306 w312] -> w254
          tunnel: w253 -> [w257 w260 w270 w282 w285 w295 w306 w312]
          tunnel: w249 -> [_ _ _ w272 _ _ _ _]
          event Timeout {
            n154 = event-data() -> ()  [unwired: 1 in, 3 out]
            n155 = call "Add State to Queue.vi"("State(s) In (\"\")"=w259) -> ("States Out"=w258:string)  [unwired: 14 in]
          }
          event "校准模式": Value Change {
            n156 = event-data() -> ()  [unwired: 1 in, 6 out]
            n157 = call "Add State to Queue.vi"("State(s) In (\"\")"=w263, "State(s) At Back (\"\")"="init: all\nidle" ("State(s) In (\"\")")) -> ("States Out"=w262:string)  [unwired: 13 in]
          }
          event "电极零点", "电极斜率", "大气压补偿", "标液1", "标液2", "滤波设定": Mouse Down {
            n158 = event-data() -> ("CtlRef"=w267:refnum<vi>)  [unwired: 1 in, 7 out]
            n159 = property class="DigNum (严格)"(reference=w267) -> (reference out=w264:refnum<vi>, "Value"=w265:dbl)  [unwired: 1 in, 1 out]
            n160 = call "数字键盘.vi"("OldNumber"=w265) -> ("NewNumber"=w266:dbl)  [unwired: 1 in]
            n161 = property class="DigNum (严格)"(reference=w264, "Val(Sgnl)"=w266) -> ()  [unwired: 1 in, 2 out]
            n162 = call "Add State to Queue.vi"("State(s) In (\"\")"=w268) -> ("States Out"=w269:string)  [unwired: 14 in]
          }
          event "电极零点", "电极斜率": Value Change {
            n163 = event-data() -> ()  [unwired: 1 in, 6 out]
            n164 = local read "电极斜率"() -> (w278:dbl)
            n165 = local read "电极零点"() -> (w277:dbl)
            n166 = global read "多参数全局变量.vi" "MB session in"() -> (w276:refnum<class "MB_Master.lvclass">)
            n167 = Bundle By Name(cluster=cluster{"K":sgl, "B":sgl} {"K"=0.0, "B"=0.0} ("用户校准参数"), "K"=w278, "B"=w277) -> (w279:cluster{"K":sgl, "B":sgl})
            n168 = call "禹山溶解氧_设置用户校准参数.vi"("用户校准参数"=w279, "MB session in"=w276) -> ("error out"=w275:errorcluster)  [unwired: 8 in, 1 out]
            n169 = Enqueue Element At Opposite End(queue=w272, element=T1."DO" ("元素"), error in (no error)=w275) -> (error out=w273:errorcluster)  [unwired: 1 in, 2 out]
            n170 = call "Add State to Queue.vi"("State(s) In (\"\")"=w274) -> ("States Out"=w281:string)  [unwired: 14 in]
          }
          event "标液1", "标液2", "大气压补偿", "盐度补偿", "盐度自动获取", "滤波设定": Value Change {
            n171 = event-data() -> ()  [unwired: 1 in, 6 out]
            n172 = flat-sequence {
              frame #0 {
                n173 = global read "断电保存变量.vi" "滤波设置"() -> (w288:T3)
                n174 = local read "盐度自动获取"() -> (w289:bool)
                n175 = local read "滤波设定"() -> (w286:dbl)
                n176 = global write "断电保存变量.vi" "盐度补偿"("盐度补偿") -> ()
                n177 = global write "断电保存变量.vi" "DO标液1"("标液1") -> ()
                n178 = global write "断电保存变量.vi" "DO标液2"("标液2") -> ()
                n179 = global write "断电保存变量.vi" "大气压补偿"("大气压补偿") -> ()
                n180 = Bundle By Name(cluster=w288, "DO"=w286) -> (w287:T3)
                n181 = global write "断电保存变量.vi" "盐度自动获取"(w289) -> ()
                n182 = global write "断电保存变量.vi" "滤波设置"(w287) -> ()
              }
              frame #1 {
                n183 = call "配置文件保存.vi"() -> ()  [unwired: 12 in]
              }
            }
            n184 = call "Add State to Queue.vi"("State(s) In (\"\")"=w283) -> ("States Out"=w284:string)  [unwired: 14 in]
          }
          event "盐度补偿": Mouse Down {
            n185 = event-data() -> ("CtlRef"=w297:refnum<vi>)  [unwired: 1 in, 7 out]
            n186 = local read "盐度自动获取"() -> (w298:bool)
            n187 = case shown="假" w298 {
              tunnel: w297 -> [w299 _]
              frame False {
                n188 = property class="DigNum (严格)"(reference=w299) -> (reference out=w300:refnum<vi>, "Value"=w301:dbl)  [unwired: 1 in, 1 out]
                n189 = call "数字键盘.vi"("OldNumber"=w301) -> ("NewNumber"=w302:dbl)  [unwired: 1 in]
                n190 = property class="DigNum (严格)"(reference=w300, "Val(Sgnl)"=w302) -> ()  [unwired: 1 in, 2 out]
              }
              frame True {
              }
            }
            n191 = call "Add State to Queue.vi"("State(s) In (\"\")"=w294) -> ("States Out"=w296:string)  [unwired: 14 in]
          }
          event "校准启动": Value Change {
            n192 = event-data() -> ()  [unwired: 1 in, 6 out]
            n193 = global read "多参数全局变量.vi" "校准运行状态"() -> (w304:T6)
            n194 = Bundle By Name(cluster=w304, "DO"=TRUE) -> (w305:T6)
            n195 = call "Add State to Queue.vi"("State(s) In (\"\")"=w309, "State(s) At Back (\"\")"="init: all\nCal: Place standard solution\n Cal: Calibration process\nidle" ("State(s) In (\"\")")) -> ("States Out"=w308:string)  [unwired: 13 in]
            n196 = global write "多参数全局变量.vi" "校准运行状态"(w305) -> ()
          }
          event "校准停止": Value Change {
            n197 = event-data() -> ()  [unwired: 1 in, 6 out]
            n198 = call "Add State to Queue.vi"("State(s) In (\"\")"="init: all\nCal: Over\nidle" ("State(s) In (\"\")")) -> ("States Out"=w311:string)  [unwired: 14 in]
          }
        }
      }
    }
  }
